vi "libtiff3_write_tiff page 16bit.vi"(0 "Handle":i32, 1 "Image Pixels (U16)":u16[][](array[numeric]), 2 "Reset":bool, 3 "Channel to process":enum16{"Red", "Green"}(ring), 4 "ImageDescription":string, 5 "error in (no error)":errorcluster, 6 "page":u32, 7 "x.pixels":i32, 8 "totalpages":i32, 9 "y.pixels":i32) -> (14 "Handle out":i32, 19 "error out":errorcluster)   [LabVIEW 2013]
doc: "SciScan 1.0 151216\nWrite a SGL (32-bit IEEE) page using LIBTIFFwriteScanLine to a file previously open for writing"
uses:
  OS Software/Source Code/support/Libtiff3/DLLs/libtiff3 (32).dll
panel:
  out "status_compression":i32
  out "status width":i32
  out "status_length":i32
  out "status_spp":i32
  out "status_bps":i32
  out "status_orientation":i32
  out "status_planarconfig":i32
  out "status_photo":i32
  out "status_writscanline":i32
  out "status_subfile":i32
  out "status_writedir":i32
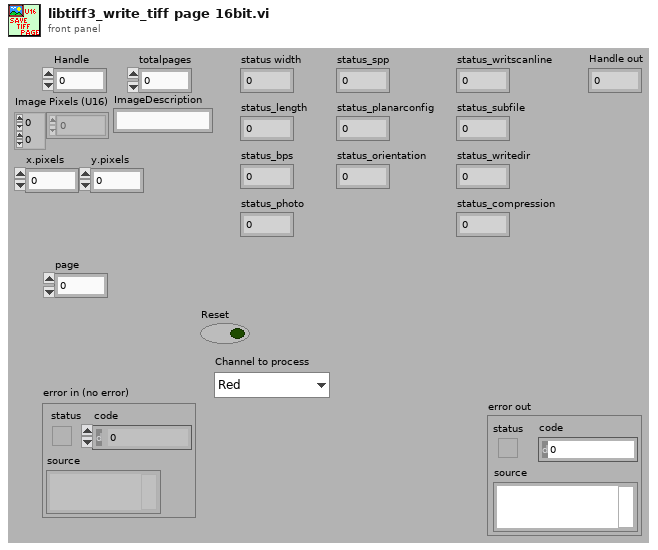
[diagram p1: front panel]
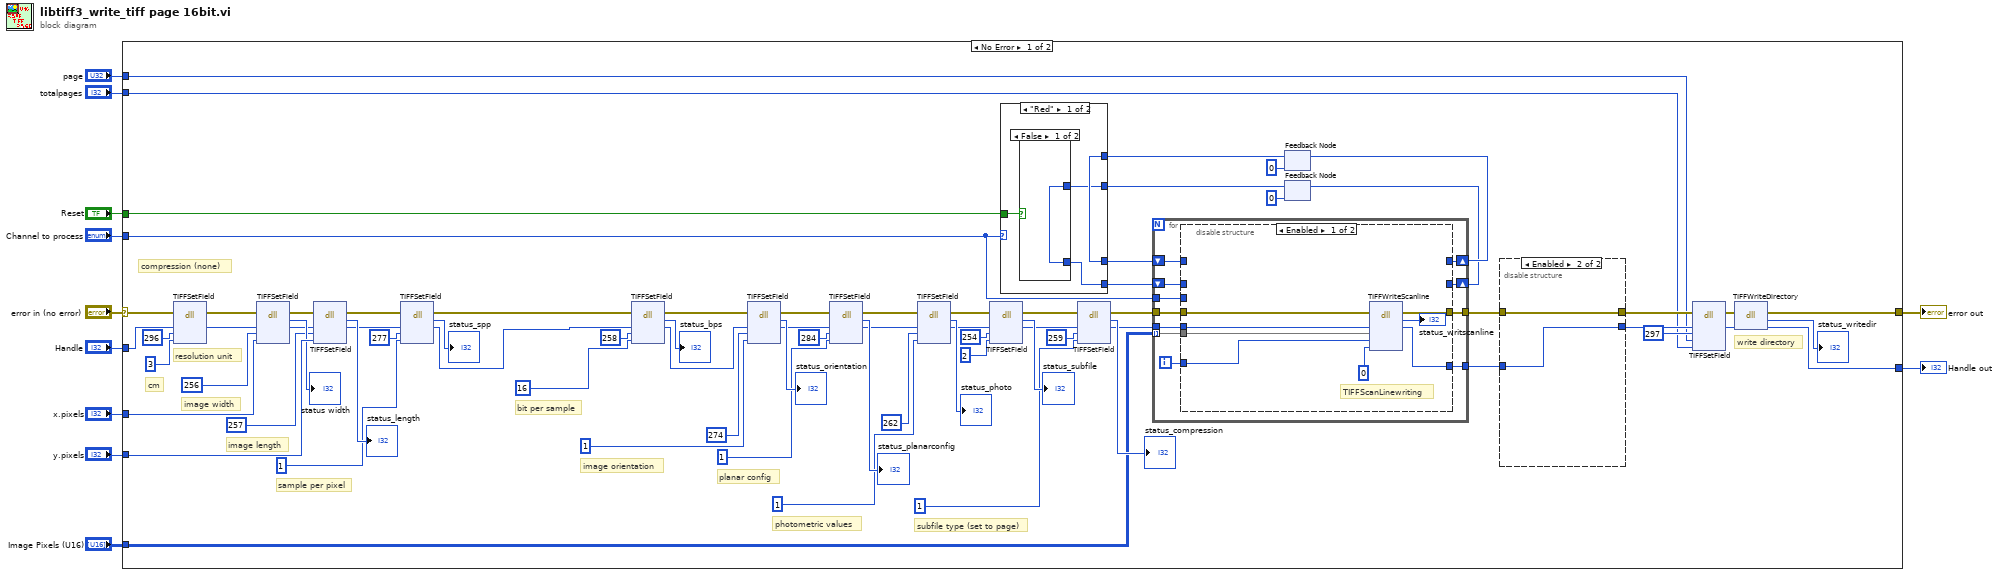
[diagram p0: block diagram]
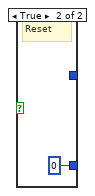
[diagram p2: hidden frame]
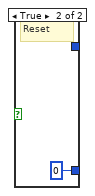
[diagram p4: hidden frame]
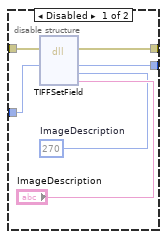
[diagram p5: hidden frame]
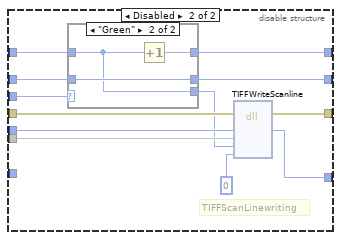
[diagram p6: hidden frame]
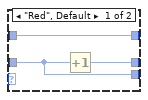
[diagram p7: hidden frame]
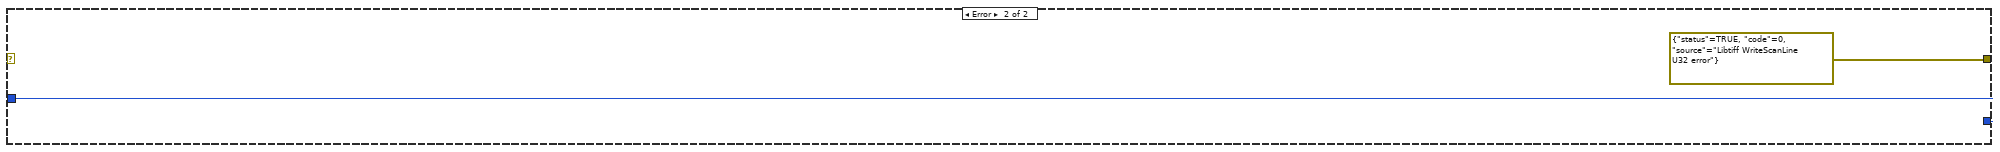
[diagram p8: hidden frame]
diagram:
  n1 = case shown="No Error" "error in (no error)" {
    selector: "error in (no error)" -> [w75 _]
    tunnel: "Handle" -> [w76 w144]
    tunnel: [w84 w144] -> w5
    tunnel: [w82 errorcluster {"status"=TRUE, "code"=0, "source"="Libtiff WriteScanLine U32 error"} ("error out")] -> w10
    tunnel: "Image Pixels (U16)" -> [w23 _]
    tunnel: "x.pixels" -> [w78 _]
    tunnel: "y.pixels" -> [w77 _]
    tunnel: "page" -> [w22 _]
    tunnel: "totalpages" -> [w24 _]
    tunnel: "Reset" -> [w17 _]
    tunnel: "Channel to process" -> [w16 _]
    frame No Error {
      # "cm"
      # "resolution unit"
      # "compression (none)"
      # "subfile type (set to page)"
      # "photometric values"
      # "planar config"
      # "image orientation"
      # "bit per sample"
      # "sample per pixel"
      # "image length"
      # "image width"
      # "write directory"
      n2 = dll-call lib="C:/OS Software/Source Code/support/Libtiff3/DLLs/libtiff3 (32).dll" fn="TIFFSetField"(error in=w75, "Handle"=w76, "TIFF_tag"=296, "value"=u32 3) -> (error out=w28:errorcluster, "Handle"=w27:i32)  [unwired: 4 in, 2 out]
      n3 = dll-call lib="C:/OS Software/Source Code/support/Libtiff3/DLLs/libtiff3 (32).dll" fn="TIFFSetField"(error in=w28, "Handle"=w27, "TIFF_tag"=256, "Value"=w78) -> (error out=w38:errorcluster, "return type"=→"status width":i32, "Handle"=w66:i32)  [unwired: 4 in, 1 out]
      n4 = dll-call lib="C:/OS Software/Source Code/support/Libtiff3/DLLs/libtiff3 (32).dll" fn="TIFFSetField"(error in=w38, "Handle"=w66, "TIFF_tag"=257, "value"=w77) -> (error out=w37:errorcluster, "return type"=→"status_length":i32, "Handle"=w63:i32)  [unwired: 4 in, 1 out]
      n5 = dll-call lib="C:/OS Software/Source Code/support/Libtiff3/DLLs/libtiff3 (32).dll" fn="TIFFSetField"(error in=w37, "Handle"=w63, "TIFF_tag"=277, "value"=u32 1) -> (error out=w26:errorcluster, "return type"=→"status_spp":i32, "Handle"=w25:i32)  [unwired: 4 in, 1 out]
      n6 = dll-call lib="C:/OS Software/Source Code/support/Libtiff3/DLLs/libtiff3 (32).dll" fn="TIFFSetField"(error in=w26, "Handle"=w25, "TIFF_tag"=258, "value"=u32 16) -> (error out=w36:errorcluster, "return type"=→"status_bps":i32, "Handle"=w58:i32)  [unwired: 4 in, 1 out]
      n7 = dll-call lib="C:/OS Software/Source Code/support/Libtiff3/DLLs/libtiff3 (32).dll" fn="TIFFSetField"(error in=w36, "Handle"=w58, "TIFF_tag"=274, "value"=u32 1) -> (error out=w35:errorcluster, "return type"=→"status_orientation":i32, "Handle"=w54:i32)  [unwired: 4 in, 1 out]
      n8 = dll-call lib="C:/OS Software/Source Code/support/Libtiff3/DLLs/libtiff3 (32).dll" fn="TIFFSetField"(error in=w35, "Handle"=w54, "TIFF_tag"=284, "value"=u32 1) -> (error out=w34:errorcluster, "return type"=→"status_planarconfig":i32, "Handle"=w50:i32)  [unwired: 4 in, 1 out]
      n9 = dll-call lib="C:/OS Software/Source Code/support/Libtiff3/DLLs/libtiff3 (32).dll" fn="TIFFSetField"(error in=w34, "Handle"=w50, "TIFF_tag"=262, "value"=u32 1) -> (error out=w33:errorcluster, "return type"=→"status_photo":i32, "Handle"=w45:i32)  [unwired: 4 in, 1 out]
      n10 = dll-call lib="C:/OS Software/Source Code/support/Libtiff3/DLLs/libtiff3 (32).dll" fn="TIFFSetField"(error in=w33, "Handle"=w45, "TIFF_tag"=254, "value"=u32 2) -> (error out=w32:errorcluster, "return type"=→"status_subfile":i32, "Handle"=w39:i32)  [unwired: 4 in, 1 out]
      n11 = dll-call lib="C:/OS Software/Source Code/support/Libtiff3/DLLs/libtiff3 (32).dll" fn="TIFFSetField"(error in=w32, "Handle"=w39, "TIFF_tag"=259, "value"=u32 1) -> (error out=w74:errorcluster, "return type"=→"status_compression":i32, "Handle"=w73:i32)  [unwired: 4 in, 1 out]
      n12 = feedback #1(0) -> (w19:i32)
      n13 = feedback #2(0) -> (w13:i32)
      n14 = case shown="\"Red\"" w16 {
        tunnel: w19 -> [w89 w95]
        tunnel: [w89 w94] -> w18
        tunnel: w17 -> [w86 w93]
        tunnel: w13 -> [w88 w92]
        tunnel: [w87 w92] -> w12
        frame "Red" {
          n15 = case shown="False" w86 {
            tunnel: [w90 0] -> w87
            tunnel: w88 -> [w90 _]
            frame False {
            }
            frame True {
              # "Reset"
            }
          }
        }
        frame "Green", Default {
          n16 = case shown="False" w93 {
            tunnel: w95 -> [w96 _]
            tunnel: [w96 0] -> w94
            frame False {
            }
            frame True {
              # "Reset"
            }
          }
        }
      }
      n17 = for {
        tunnel: [w112] -> w69
        tunnel: [w113] -> w70
        tunnel: w73 -> [w115]
        tunnel: w74 -> [w116]
        tunnel: w23 -> [w114] mode=indexing
        shift-right: [w110] -> w21
        shift-left: w18 -> [w111]
        shift-right: [w108] -> w14
        shift-left: w12 -> [w107]
        tunnel: w16 -> [w106]
        i -> [w109]
        n18 = disable-structure shown="Enabled" {
          disable-tunnel: w116 -> [w124 w136]
          disable-tunnel: w115 -> [w123 w135]
          disable-tunnel: w114 -> [w122 w134]
          disable-tunnel: [w121 w133] -> w113
          disable-tunnel: [w119 w132] -> w112
          disable-tunnel: w111 -> [_ w126]
          disable-tunnel: [_ w130] -> w110
          disable-tunnel: w109 -> [w117 _]
          disable-tunnel: w107 -> [_ w128]
          disable-tunnel: [_ w127] -> w108
          disable-tunnel: w106 -> [_ w129]
          frame Enabled {
            # "TIFFScanLinewriting"
            n19 = dll-call lib="C:/OS Software/Source Code/support/Libtiff3/DLLs/libtiff3 (32).dll" fn="TIFFWriteScanline"(error in=w124, "Handle"=w123, "buffer"=w122, "row"=w117, "sample"=0) -> (error out=w121:errorcluster, "return type"=→"status_writscanline":i32, "Handle"=w119:i32)  [unwired: 5 in, 1 out]
          }
          frame Disabled {
            # "TIFFScanLinewriting"
            n20 = case shown="\"Green\"" w129 {
              tunnel: w126 -> [w139 w140]
              tunnel: [w139 w142] -> w130
              tunnel: w128 -> [w137 w141]
              tunnel: [w138 w141] -> w127
              tunnel: [w137 w140] -> w125
              frame "Red", Default {
                n21 = Increment(x=w137) -> (x+1=w138:i32)
              }
              frame "Green" {
                n22 = Increment(x=w140) -> (x+1=w142:i32)
              }
            }
            n23 = dll-call lib="C:/OS Software/Source Code/support/Libtiff3/DLLs/libtiff3 (32).dll" fn="TIFFWriteScanline"(error in=w136, "Handle"=w135, "buffer"=w134, "row"=w125, "sample"=0) -> (error out=w133:errorcluster, "Handle"=w132:i32)  [unwired: 5 in, 2 out]
          }
        }
      }
      n24 = feedback-in #1(w21) -> ()
      n25 = feedback-in #2(w14) -> ()
      n26 = disable-structure shown="Enabled" {
        disable-tunnel: [w103 w105] -> w72
        disable-tunnel: [w102 w104] -> w71
        disable-tunnel: w70 -> [w99 w105]
        disable-tunnel: w69 -> [w98 w104]
        frame Disabled {
          w100 = 270  # ImageDescription
          n27 = dll-call lib="C:/OS Software/Source Code/support/Libtiff3/DLLs/libtiff3 (32).dll" fn="TIFFSetField"(error in=w99, "Handle"=w98, "TIFF_tag"=w100, "Value"="ImageDescription") -> (error out=w103:errorcluster, "Handle"=w102:i32)  [unwired: 4 in, 2 out]
        }
        frame Enabled {
        }
      }
      n28 = dll-call lib="C:/OS Software/Source Code/support/Libtiff3/DLLs/libtiff3 (32).dll" fn="TIFFSetField"(error in=w72, "Handle"=w71, "TIFF_tag"=297, "page"=w22, "totalpages"=w24) -> (error out=w80:errorcluster, "Handle"=w79:i32)  [unwired: 5 in, 2 out]
      n29 = dll-call lib="C:/OS Software/Source Code/support/Libtiff3/DLLs/libtiff3 (32).dll" fn="TIFFWriteDirectory"(error in=w80, "Handle"=w79) -> (error out=w82:errorcluster, "return type"=→"status_writedir":i32, "Handle"=w84:i32)  [unwired: 2 in, 1 out]
    }
    frame Error {
    }
  }
  "Handle out" <- w5
  "error out" <- w10
